vi "joy_rio.vi"() -> ()   [LabVIEW 2017]
uses:
  <vilib>/myRIO/Instrument Drivers/Onboard IO/PWM/typedefs/PWM Reference.ctl
  <vilib>/myRIO/Common/Instrument Driver Framework/Utilities/typedefs/myRIO Generic Hardware Reference.ctl
  <vilib>/myRIO/Common/Instrument Driver Framework/Utilities/typedefs/Hardware Version Enum.ctl
  <vilib>/myRIO/Common/Instrument Driver Framework/Utilities/typedefs/myRIO v1.0 Reference.ctl
  <vilib>/myRIO/Common/Instrument Driver Framework/Utilities/typedefs/Generic FPGA Reference.ctl
  <vilib>/myRIO/Common/Instrument Driver Framework/myRIO v1.0/PWM/typedefs/PWM Channels Enum.ctl
  <vilib>/myRIO/Instrument Drivers/Onboard IO/PWM/typedefs/PWM Configuration.ctl
  <vilib>/userdefined/High Color/nirio_resource_hc.ctl
  <vilib>/myRIO/Common/Instrument Driver Framework/Utilities/vis/Is FPGA Ref Available.vi
  <vilib>/myRIO/Common/Instrument Driver Framework/myRIO v1.0/PWM/vis/myRIO v1.1 Open PWM.vi
  <vilib>/myRIO/Instrument Drivers/Onboard IO/PWM/vis/Set Duty Cycle and Frequency.vi
  <vilib>/myRIO/Common/Instrument Driver Framework/myRIO v1.0/UART/vis/myRIO v1.0 Close UART.vi
  <vilib>/myRIO/Common/Instrument Driver Framework/Utilities/vis/Validate Channels.vi
  <vilib>/myRIO/Common/Instrument Driver Framework/myRIO v1.0/PWM/vis/myRIO v1.0 Reserve PWM.vi
  <vilib>/myRIO/Common/Instrument Driver Framework/myRIO v1.0/PWM/vis/myRIO v1.0 Build MUX Configuration PWM.vi
  <vilib>/myRIO/Common/Instrument Driver Framework/myRIO v1.0/Resource Manager/vis/myRIO v1.0 Reserve Channel List.vi
  <vilib>/myRIO/Common/Instrument Driver Framework/myRIO v1.0/Resource Manager/vis/myRIO v1.0 Create Configuration List.vi
  <vilib>/myRIO/Common/Instrument Driver Framework/myRIO v1.0/Resource Manager/vis/myRIO v1.0 Reserve Channel.vi
  <vilib>/myRIO/Common/Instrument Driver Framework/myRIO v1.0/Resource Manager/vis/myRIO v1.0 Unreserve Channel.vi
  <vilib>/myRIO/Common/Instrument Driver Framework/myRIO v1.0/Resource Manager/vis/myRIO v1.0 Build Mutex Name.vi
  <vilib>/myRIO/Common/Instrument Driver Framework/Utilities/vis/FPGA Ref Manager.vi
  <vilib>/myRIO/Common/Instrument Driver Framework/myRIO v1.0/myRIO v1.0 Reset FPGA.vi
  <vilib>/myRIO/Common/Instrument Driver Framework/myRIO v1.0/IRQ/vis/myRIO v1.0 IRQ Info FGV.vi
  <vilib>/myRIO/Common/Instrument Driver Framework/myRIO v1.0/IRQ/vis/myRIO v1.0 Timer IRQ Info FGV.vi
  <vilib>/myRIO/Common/Instrument Driver Framework/myRIO v1.0/IRQ/vis/myRIO v1.0 ISR Agent.vi
  <vilib>/Utility/VariantDataType/GetNumericInfo.vi
  <vilib>/Utility/error.llb/Error Cluster From Error Code.vi
  <vilib>/myRIO/Common/Instrument Driver Framework/myRIO v1.0/myRIO v1.1 Open.vi
  <vilib>/myRIO/Common/Instrument Driver Framework/Utilities/vis/IO Manager.vi
  <vilib>/myRIO/Common/Instrument Driver Framework/Utilities/vis/Configuration Manager.vi
  <vilib>/myRIO/Common/Instrument Driver Framework/myRIO v1.0/Resource Manager/vis/myRIO v1.0 Configure IO.vi
  <vilib>/myRIO/Common/Instrument Driver Framework/myRIO v1.0/myRIO v1.0 Close.vi
  <vilib>/myRIO/Common/Instrument Driver Framework/myRIO v1.0/PWM/vis/myRIO v1.0 Write PWM.vi
  <vilib>/myRIO/Express VI/Onboard IO/PWM/PWM Express VI.xnode
  <vilib>/myRIO/Instrument Drivers/Onboard IO/PWM/vis/myRIO PWM Open.xnode
  <vilib>/myRIO/Instrument Drivers/Onboard IO/PWM/PWM.lvlib
  <vilib>/myRIO/Instrument Drivers/Utilities/Utilities.lvlib
panel:
  in  "stop":bool
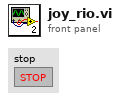
[diagram p1: front panel]
types:
  T1 = typedef "PWM.lvlib/PWM Reference.ctl" = cluster{"myRIO Reference":T2, "PWM Channels Enum":T6, "PWM Configuration":T7}
  T2 = typedef "myRIO Generic Hardware Reference.ctl" = cluster{"myRIO Model":T3, "myRIO Hardware Reference":T4}
  T3 = typedef "Hardware Version Enum.ctl" = enum16{"Unknown", "myRIO-1900", "myRIO-1950", "roboRIO", "NI ELVIS RIO CM"}
  T4 = typedef "myRIO v1.0 Reference.ctl" = cluster{"Generic FPGA Reference":T5, "Allow multiple opens":bool}
  T5 = typedef "Generic FPGA Reference.ctl" = refnum<k20>
  T6 = typedef "PWM Channels Enum.ctl" = enum16{"Not Connected", "C/PWM0", "C/PWM1", "A/PWM0", "A/PWM1", "A/PWM2", "B/PWM0", "B/PWM1", "B/PWM2", "PWM/PWM0", "PWM/PWM1", "PWM/PWM2", "PWM/PWM3", "PWM/PWM4", "PWM/PWM5", "PWM/PWM6", "PWM/PWM7", "PWM/PWM8", "PWM/PWM9"}
  T7 = typedef "PWM.lvlib/PWM Configuration.ctl" = cluster{"Frequency":dbl, "Duty Cycle":dbl}
  T8 = typedef "nirio_resource_hc.ctl" = tag
  T9 = cluster{"Array of Boolean[0]":bool, "Array of Boolean[1]":bool, "Array of Boolean[2]":bool, "Array of Boolean[3]":bool, "Array of Boolean[4]":bool, "Array of Boolean[5]":bool, "Array of Boolean[6]":bool, "Array of Boolean[7]":bool, "Array of Boolean[8]":bool}
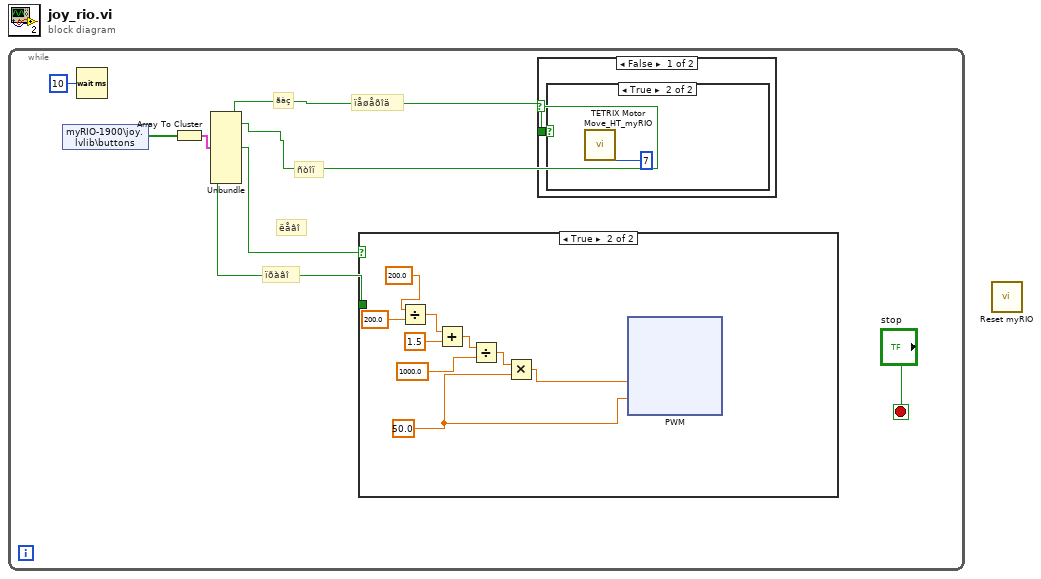
[diagram p0: block diagram]
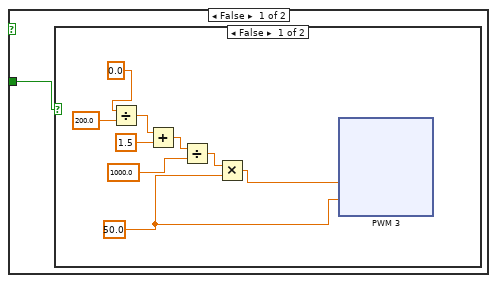
[diagram p2: hidden frame]
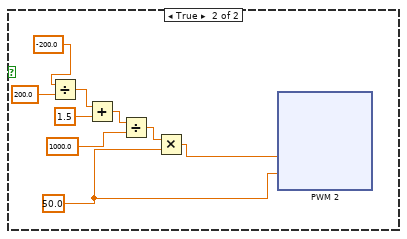
[diagram p3: hidden frame]
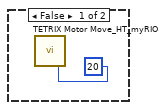
[diagram p4: hidden frame]
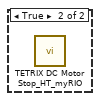
[diagram p5: hidden frame]
diagram:
  n1 = while {
    stop <- "stop" stop-if-true
    # "ïðàâî"
    # "ëåâî"
    # "ñòîï"
    # "ïåøåõîä"
    # "ãàç"
    n2 = shared-variable "myRIO-1900\\joy.lvlib\\buttons"() -> (w6:bool[])  [unwired: 1 in, 1 out]
    n3 = Wait (ms)(milliseconds to wait=u32 10) -> ()  [unwired: 1 out]
    n4 = Array To Cluster(array=w6) -> (cluster=w7:T9)
    n5 = Unbundle(w7) -> ("Array of Boolean[0]"=w3:bool, "Array of Boolean[1]"=w5:bool, "Array of Boolean[4]"=w2:bool, "Array of Boolean[5]"=w1:bool)  [unwired: 5 out]
    n6 = case shown="True" w2 {
      tunnel: w1 -> [w9 _]
      frame False {
        n7 = case shown="False" w9 {
          frame False {
            w11 = sgl 50.0 ("y")
            n8 = Divide(x=sgl 0.0, y=sgl 200.0) -> (x/y=w17:sgl)
            n9 = Add(x=w17, y=sgl 1.5) -> (x+y=w16:sgl)
            n10 = Divide(x=w16, y=sgl 1000.0) -> (x/y=w15:sgl)
            n11 = Multiply(x=w15, y=w11) -> (x*y=w18:sgl)
            n12 = xnode "PWM 3"("Duty Cycle"=w18, "Frequency [Hz]"=w11) -> ()  [unwired: 1 in, 1 out]
          }
          frame True {
            w55 = sgl 50.0 ("y")
            n13 = Divide(x=sgl -200.0, y=sgl 200.0) -> (x/y=w61:sgl)
            n14 = Add(x=w61, y=sgl 1.5) -> (x+y=w60:sgl)
            n15 = Divide(x=w60, y=sgl 1000.0) -> (x/y=w59:sgl)
            n16 = Multiply(x=w59, y=w55) -> (x*y=w62:sgl)
            n17 = xnode "PWM 2"("Duty Cycle"=w62, "Frequency [Hz]"=w55) -> ()  [unwired: 1 in, 1 out]
          }
        }
      }
      frame True {
        w99 = sgl 50.0 ("y")
        n18 = Divide(x=sgl 200.0, y=sgl 200.0) -> (x/y=w105:sgl)
        n19 = Add(x=w105, y=sgl 1.5) -> (x+y=w104:sgl)
        n20 = Divide(x=w104, y=sgl 1000.0) -> (x/y=w103:sgl)
        n21 = Multiply(x=w103, y=w99) -> (x*y=w106:sgl)
        n22 = xnode "PWM"("Duty Cycle"=w106, "Frequency [Hz]"=w99) -> ()  [unwired: 1 in, 1 out]
      }
    }
    n23 = case shown="False" w5 {
      tunnel: w3 -> [w142 _]
      frame False {
        n24 = case shown="True" w142 {
          frame False {
            n25 = call <vilib>:"TETRIX Motor Move_HT_myRIO.vi"("Power (-100 to 100)\n0 = Stop/Brake\n-128 = Stop/Coast"=i8 20 ("Power (-100 to 100)\n0 = Stop/Brake\n-128 = Stop/Coast")) -> ()  [unwired: 6 in, 1 out]
          }
          frame True {
            n26 = call <vilib>:"TETRIX Motor Move_HT_myRIO.vi"("Power (-100 to 100)\n0 = Stop/Brake\n-128 = Stop/Coast"=i8 7 ("Power (-100 to 100)\n0 = Stop/Brake\n-128 = Stop/Coast")) -> ()  [unwired: 6 in, 1 out]
          }
        }
      }
      frame True {
        n27 = call <vilib>:"TETRIX DC Motor Stop_HT_myRIO.vi"() -> ()  [unwired: 4 in, 1 out]
      }
    }
  }
  n28 = call <vilib>:"Reset myRIO.vi"() -> ()  [unwired: 11 in, 1 out]
